vi "Set Command Timeout.vi"(4 "error in":errorcluster, 6 "CommandTimeout":i32=30, 7 "Connection In":refnum<k7>) -> (0 "error out":errorcluster, 3 "Connection Out":refnum<k7>)   [LabVIEW 2014, in "hse-db.lvlib" / "ADO-DB-Driver.lvlib"]
uses:
  ADO-DB-Driver.lvlib
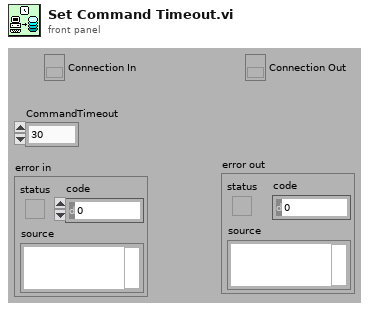
[diagram p1: front panel]
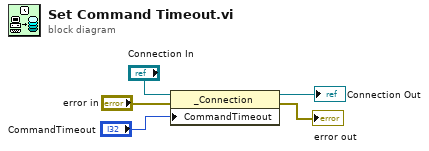
[diagram p0: block diagram]
diagram:
  n1 = property class="_Connection"(reference="Connection In", error in="error in", "CommandTimeout"="CommandTimeout") -> (reference out=→"Connection Out":refnum<k7>, error out=→"error out":errorcluster)
